vi "neardevice_cap_navigation.vi"() -> ()   [LabVIEW 2010]
uses:
  <userlib>/Nanonis Prog Interface V5/Nanonis Prog Interface.lvlib
panel:
  in  "# of Averages":dbl
  in  "milliseconds to wait":u32
  in  "stop":bool
  in  "?":bool
  in  "Max Steps":u16=500
  in  "Direction":enum16{"X +", "X -", "Y +", "Y -", "Z +", "Z -"}(ring)
  out "Delta":cluster{"index":i32, sgl}[](graph)
  in  "Number of Steps":u16=500
  out "Capacitance":cluster{"index":i32, sgl}[](graph)
  in  "Frequency (Hz)":sgl=250.0
  in  "Amplitude (V)":sgl=150.0
  # "Max Steps On"
  # "Max Steps Off"
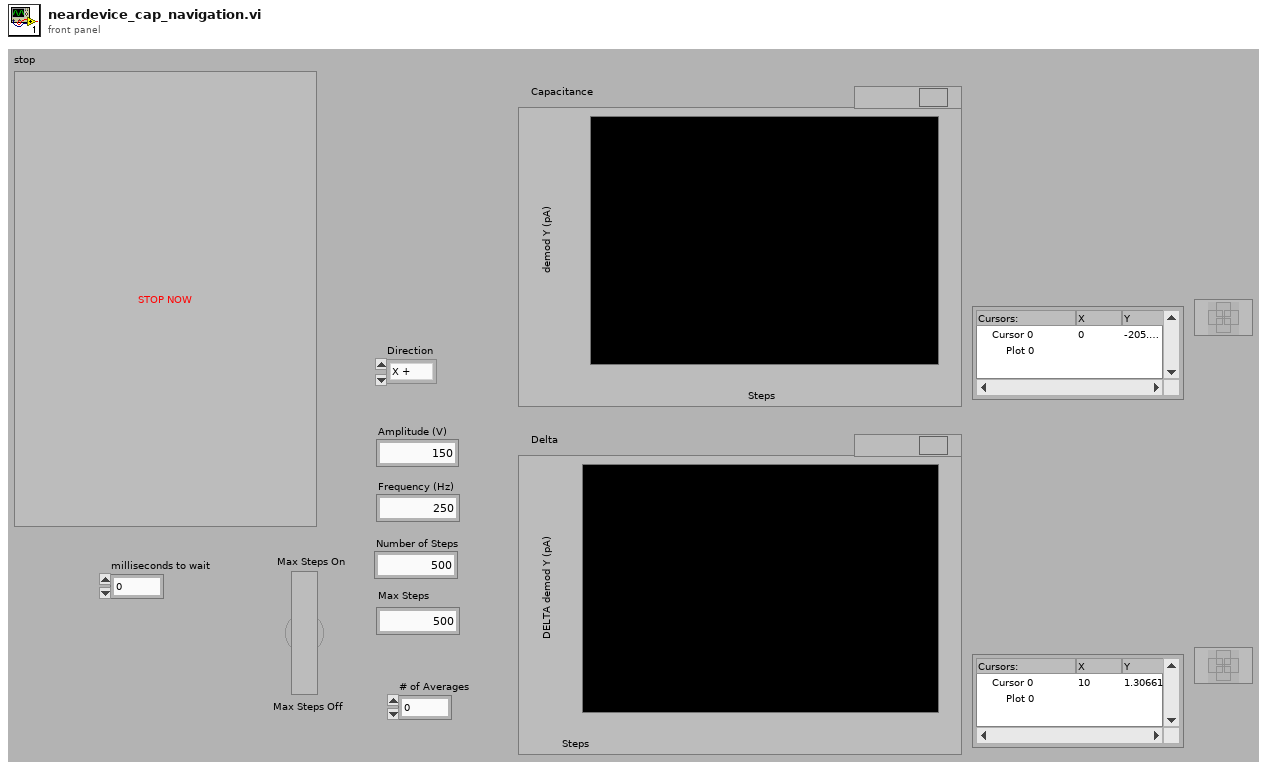
[diagram p1: front panel]
types:
  T1 = enum8{"Group 1", "Group 2", "Group 3", "Group 4", "Group 5", "Group 6"}
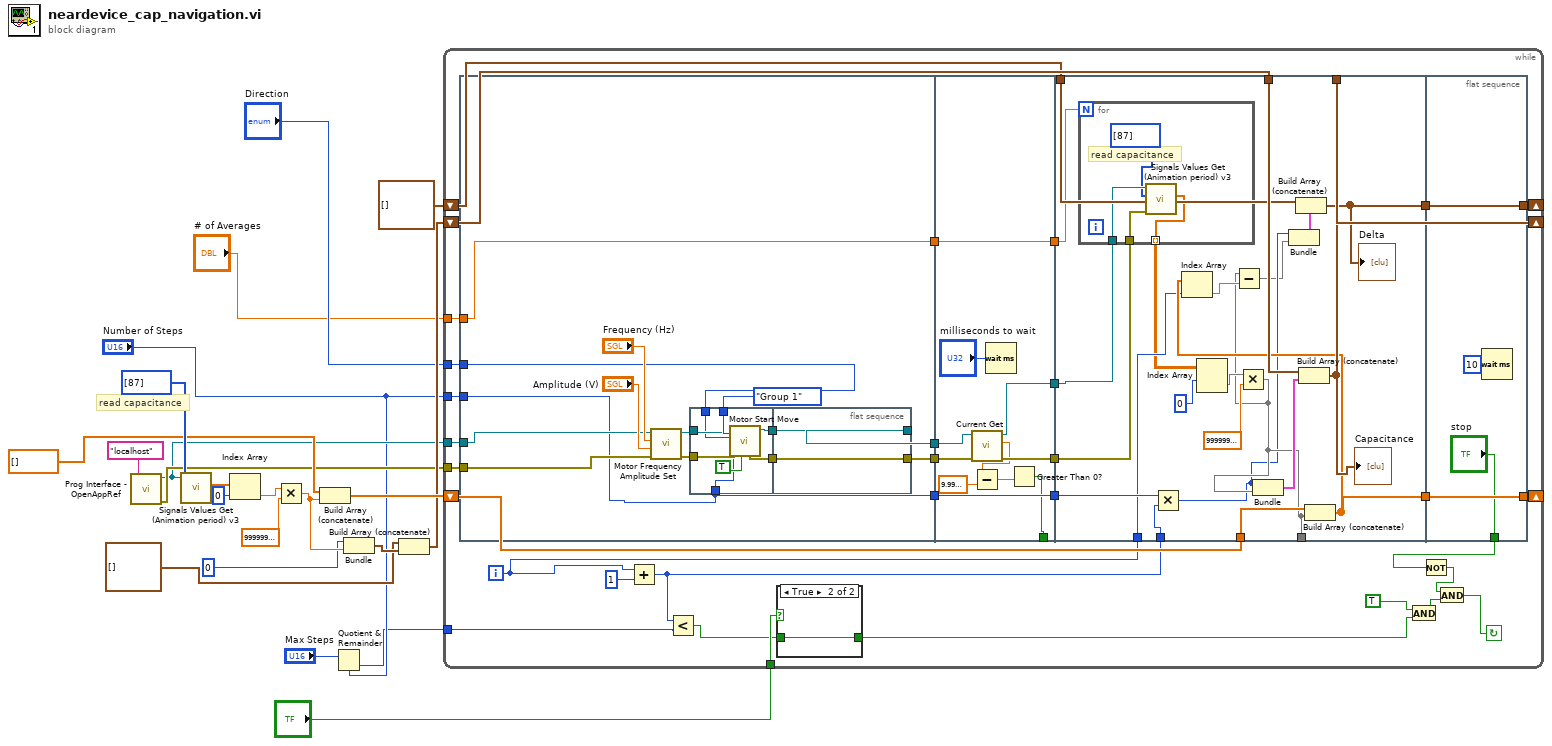
[diagram p0: block diagram]
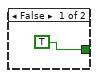
[diagram p2: hidden frame]
diagram:
  # "read capacitance"
  n1 = call <userlib>:"Prog Interface - OpenAppRef.vi"("Machine name (local machine IP)"="localhost" ("machine name (localhost)")) -> ("Error out"=w9:errorcluster, "Application reference"=w8:refnum<vi>)  [unwired: 5 in]
  n2 = call <userlib>:"Signals Values Get (Animation period) v3.vi"("Signals indexes (0-127)"=i8[] [87], "Application ref in"=w8) -> ("Signals Values"=w19:sgl[])  [unwired: 6 in, 2 out]
  n3 = Index Array(array=w19, index=0) -> (element=w18:sgl)
  n4 = Multiply(x=w18, y=sgl 1000000000000.0) -> (x*y=w14:sgl)
  n5 = Build Array (concatenate)(sgl[] [], w14) -> (w15:sgl[])
  n6 = Quotient & Remainder(x="Max Steps", y="Number of Steps") -> (floor(x/y)=w3:u16)  [unwired: 1 out]
  n7 = Bundle("index"=0, w14) -> (w12:cluster{"index":i32, sgl})  [unwired: 1 in]
  n8 = Build Array (concatenate)(cluster{i32, sgl}[] [], w12) -> (w11:cluster{"index":i32, sgl}[])
  n9 = while {
    shift-right: [w53] -> _
    shift-left: w11 -> [w52]
    shift-right: [w51] -> _
    shift-left: w15 -> [w50]
    tunnel: w8 -> [w47]
    tunnel: w9 -> [w46]
    shift-right: [w40] -> _
    shift-left: cluster{i32, sgl}[] [] -> [w39]
    tunnel: "Direction" -> [w38]
    tunnel: "Number of Steps" -> [w37]
    tunnel: w3 -> [w30]
    tunnel: "?" -> [w36]
    tunnel: "# of Averages" -> [w25]
    i -> [w33]
    stop <- w27 continue-if-true
    n10 = flat-sequence {
      tunnel: [w60] -> w55
      tunnel: w47 -> [w63]
      tunnel: w46 -> [w66]
      tunnel: [w65] -> w45
      tunnel: [w64] -> w44
      tunnel: w38 -> [w59]
      tunnel: w37 -> [w60]
      tunnel: w25 -> [w58]
      tunnel: [w58] -> w24
      tunnel: w55 -> [w92]
      tunnel: [w92] -> w54
      tunnel: w45 -> [w91]
      tunnel: w44 -> [w90]
      tunnel: [w89] -> w43
      tunnel: [w88] -> w42
      tunnel: [w85] -> _
      tunnel: w24 -> [w82]
      tunnel: [w82] -> w23
      tunnel: [w109] -> w53
      tunnel: w31 -> [w111]
      tunnel: w54 -> [w106]
      tunnel: w52 -> [w108]
      tunnel: w50 -> [w107]
      tunnel: [w102] -> _
      tunnel: [w105] -> w49
      tunnel: w43 -> [w94]
      tunnel: w42 -> [w95]
      tunnel: w33 -> [w104]
      tunnel: [w98] -> w41
      tunnel: w39 -> [w99]
      tunnel: w23 -> [w96]
      tunnel: [w122] -> w51
      tunnel: w49 -> [w122]
      tunnel: w41 -> [w120]
      tunnel: [w120] -> w40
      tunnel: ["stop"] -> w26
      frame #0 {
        n11 = call <userlib>:"Motor Frequency Amplitude Set.vi"("Error in (no error)"=w66, "Amplitude (V) (NaN=no change)"="Amplitude (V)", "Frequency (Hz) (NaN=no change)"="Frequency (Hz)", "Application ref in"=w63) -> ("Error out"=w67:errorcluster, "Application ref out"=w68:refnum<vi>)  [unwired: 6 in]
        n12 = flat-sequence {
          tunnel: T1."Group 1" ("Group") -> [w78]
          tunnel: w68 -> [w77]
          tunnel: w67 -> [w76]
          tunnel: w60 -> [w75]
          tunnel: [w74] -> w62
          tunnel: [w73] -> w61
          tunnel: w59 -> [w72]
          tunnel: [w80] -> w64
          tunnel: [w81] -> w65
          tunnel: w62 -> [w81]
          tunnel: w61 -> [w80]
          frame #0 {
            n13 = call <userlib>:"Motor Start Move.vi"("Wait until finished? (F)"=TRUE, "Group"=w78, "Error in (no error)"=w76, "Number of steps"=w75, "Direction"=w72, "Application ref in"=w77) -> ("Error out"=w73:errorcluster, "Application ref out"=w74:refnum<vi>)  [unwired: 3 in]
          }
          frame #1 {
          }
        }
      }
      frame #1 {
        n14 = call <userlib>:"Current Get.vi"("Error in (no error)"=w90, "Application ref in"=w91) -> ("Error out"=w89:errorcluster, "Current (A)"=w87:sgl, "Application ref out"=w88:refnum<vi>)  [unwired: 5 in]
        n15 = Subtract(x=w87, y=sgl 1e-09) -> (x-y=w86:sgl)
        n16 = Wait (ms)(milliseconds to wait="milliseconds to wait") -> ()  [unwired: 1 out]
        n17 = Greater Than 0?(x=w86) -> (x > 0?=w85:bool)
      }
      frame #2 {
        n18 = for {
          N: w96 -> [_]
          tunnel: w95 -> [w118]
          tunnel: w94 -> [w117]
          tunnel: [w115] -> w93 mode=indexing
          # "read capacitance"
          n19 = call <userlib>:"Signals Values Get (Animation period) v3.vi"("error in (no error)"=w117, "Signals indexes (0-127)"=i8[] [87], "Application ref in"=w118) -> ("Signals Values"=w115:sgl[])  [unwired: 5 in, 2 out]
        }
        n20 = Multiply(x=w106, y=w111) -> (x*y=w101:i32)
        n21 = Index Array(array=w93, index (row)=0 ("index")) -> (element=w113:sgl[])  [unwired: 1 in]
        n22 = Multiply(x=w113, y=sgl 1000000000000.0) -> (x*y=w102:sgl[])
        n23 = Bundle(w101, w102) -> (w110:cluster{i32, sgl[]})  [unwired: 1 in]
        n24 = Build Array (concatenate)(w108, w110) -> (w109:cluster{"index":i32, sgl}[])
        "Capacitance" <- w109
        n25 = Build Array (concatenate)(w107, w102) -> (w105:sgl[])
        n26 = Index Array(array=w105, index=w104) -> (element=w103:sgl)
        n27 = Subtract(x=w102, y=w103) -> (x-y=w97:sgl[])
        n28 = Bundle(w101, w97) -> (w100:cluster{i32, sgl[]})  [unwired: 1 in]
        n29 = Build Array (concatenate)(w99, w100) -> (w98:cluster{i32, sgl}[])
        "Delta" <- w98
      }
      frame #3 {
        n30 = Wait (ms)(milliseconds to wait=u32 10) -> ()  [unwired: 1 out]
      }
    }
    n31 = Add(x=w33, y=u16 1) -> (x+y=w31:i32)
    n32 = Less?(x=w31, y=w30) -> (x < y?=w32:bool)
    n33 = case shown="True" w36 {
      tunnel: w32 -> [_ w57]
      tunnel: [TRUE w57] -> w34
      frame False {
      }
      frame True {
      }
    }
    n34 = And(x=TRUE, y=w34) -> (x .and. y?=w28:bool)
    n35 = Not(x=w26) -> (.not. x?=w29:bool)
    n36 = And(x=w29, y=w28) -> (x .and. y?=w27:bool)
  }
